vi "Event Handler.vi"(8 "error in":errorcluster, 11 "Listbox in":refnum<class "Multi Column Listbox.lvclass">) -> (0 "error out":errorcluster, 3 "Listbox out":refnum<class "Multi Column Listbox.lvclass">)   [LabVIEW 2013, in "Table Manager.lvlib" / "Multi Column Listbox.lvclass"]
doc: "Contains a loop and event structure to handle all common MCLB user interactions."
uses:
  Multi Column Listbox.lvclass
  Table Manager.lvlib
  <vilib>/Utility/miscctls.llb/LVPositionTypeDef.ctl
  Table Manager/Menu Select.ctl
  Table Manager/Table Manager.lvclass
  <vilib>/Utility/miscctls.llb/LVRowAndColumnTypeDef.ctl
panel:
  out "Char":i16
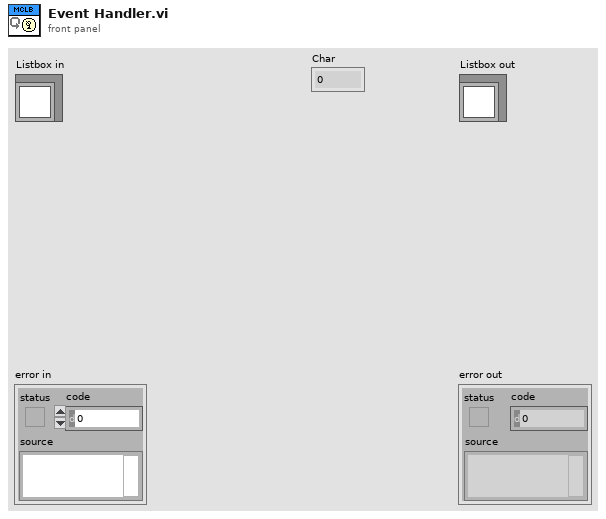
[diagram p1: front panel]
types:
  T1 = typedef "LVPositionTypeDef.ctl" = cluster{"Left":i32, "Top":i32}
  T2 = typedef "LVRowAndColumnTypeDef.ctl" = cluster{"Row":i32, "Column":i32}
  T3 = typedef "Table Manager.lvlib/Table Manager.lvclass/Menu Select.ctl" = cluster{"Line Name":string, "Selected Value":string, "Row":i32, "Column":i32, "Table Index":i32}
  T4 = typedef "Table Manager.lvlib/Table Manager.lvclass/object ref.ctl" = cluster{"engine":refnum<data-value>, "Node Ref":refnum<data-value>}
  T5 = typedef "NISE_CEF_Node.lvclass/RefreshUIEvent.ctl" = refnum<user-event>
  T6 = typedef "Table Manager.lvlib/Multi Column Listbox.lvclass/Int Reg Events.ctl" = refnum<event-registration>
  T7 = typedef "control module editor.lvclass/dialog output action.ctl" = enum16{"Tag Created", "Tag Selected", "Set Default", "disconnect"}
  T8 = typedef "LVPoint32TypeDef.ctl" = cluster{"Horizontal":i32, "Vertical":i32}
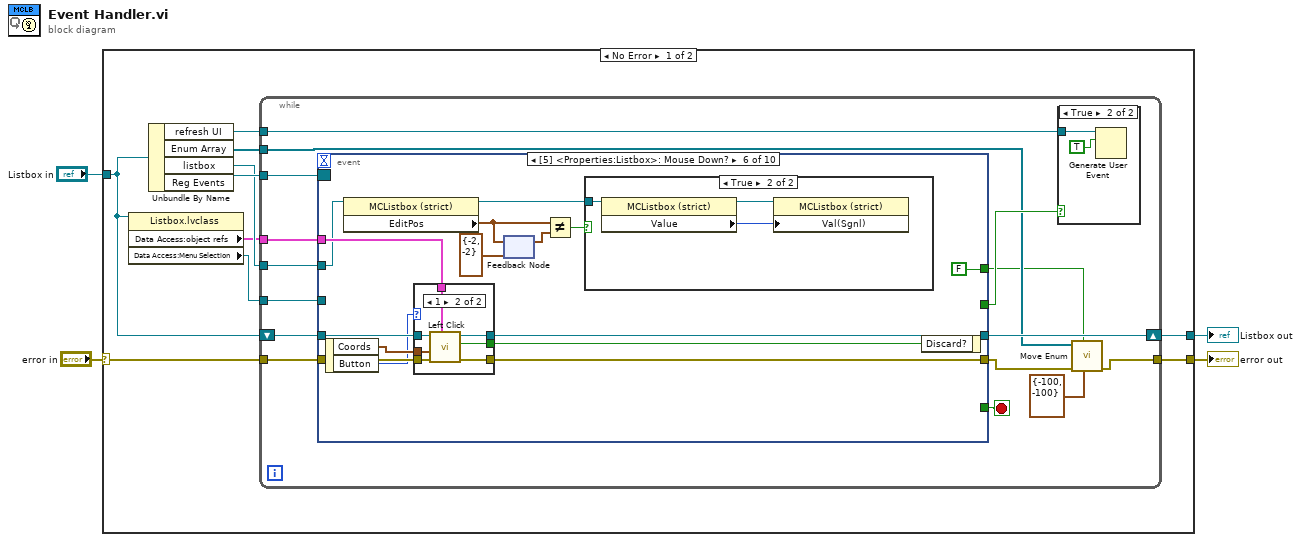
[diagram p0: block diagram]
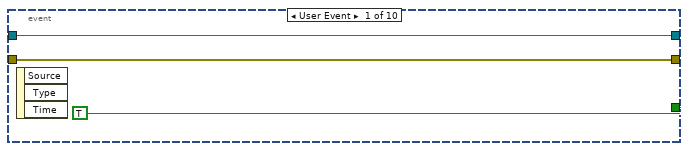
[diagram p3: hidden frame]
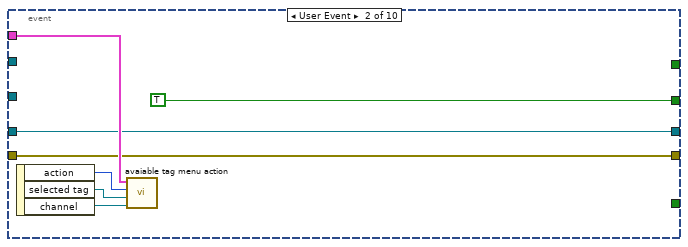
[diagram p4: hidden frame]
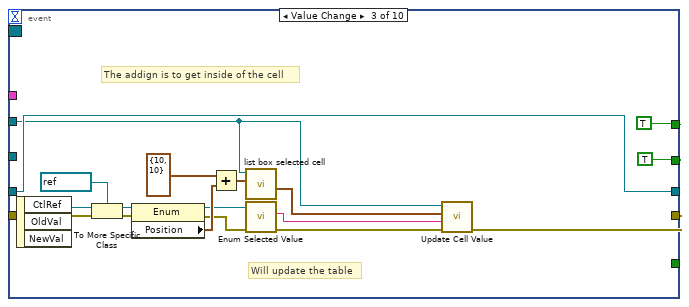
[diagram p5: hidden frame]
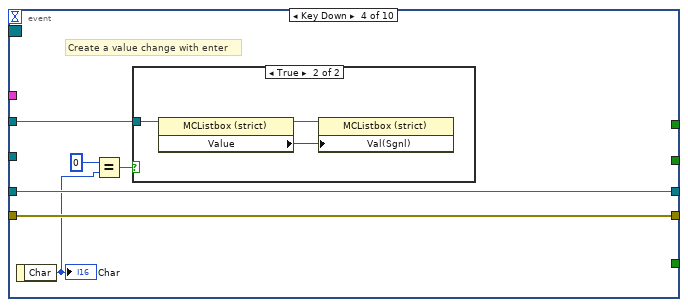
[diagram p6: hidden frame]
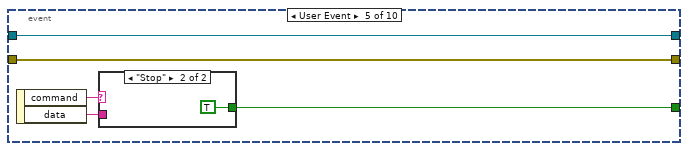
[diagram p8: hidden frame]
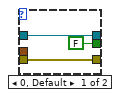
[diagram p11: hidden frame]
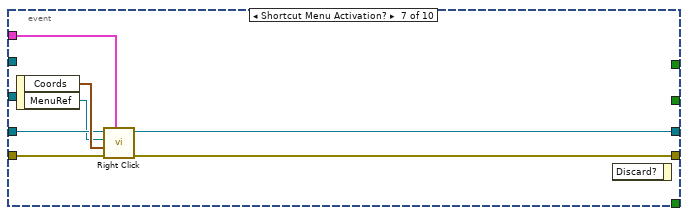
[diagram p12: hidden frame]
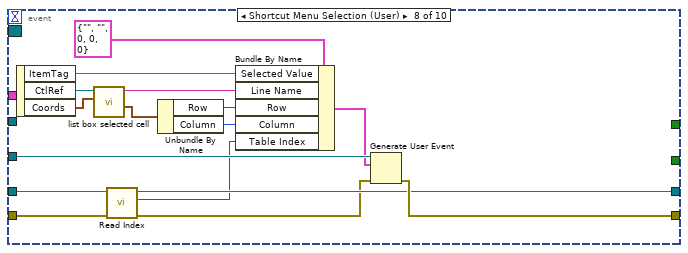
[diagram p13: hidden frame]
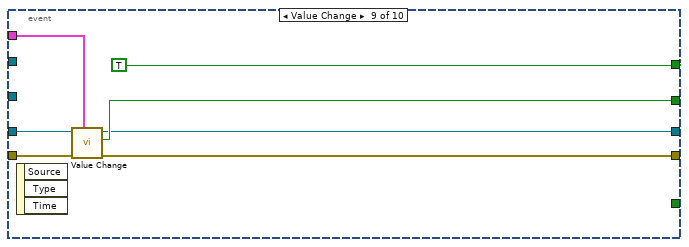
[diagram p14: hidden frame]
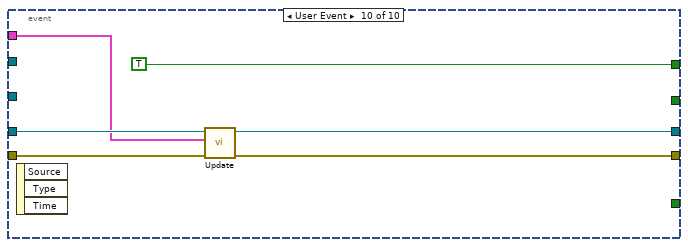
[diagram p15: hidden frame]
diagram:
  n1 = case shown="No Error" "error in" {
    selector: "error in" -> [w12 w140]
    tunnel: [w11 w140] -> w2
    tunnel: [w14 w139] -> w3
    tunnel: "Listbox in" -> [w7 w139]
    frame No Error {
      n2 = property class="Listbox.lvclass"(reference=w7) -> ("Data Access:object refs"=w6:T4, "Data Access:Menu Selection"=w5:refnum<user-event>)  [unwired: 1 in, 2 out]
      n3 = Unbundle By Name(w7) -> ("refresh UI"=w9:T5, "Enum Array"=w8:refnum<vi>[], "listbox"=w10:refnum<vi>, "Reg Events"=w13:T6)
      n4 = while {
        shift-right: [w25] -> w14
        shift-left: w7 -> [w26]
        tunnel: w13 -> [w28]
        tunnel: w6 -> [w27]
        tunnel: w12 -> [w24]
        tunnel: [w20] -> w11
        tunnel: w8 -> [w22]
        tunnel: w10 -> [w19]
        tunnel: w9 -> [w18]
        tunnel: w5 -> [w15]
        stop <- w29 stop-if-true
        n5 = event shown="[5] <Properties:Listbox>: Mouse Down?" {
          selector: w28 -> [_ _ _ _ _ _ _ _ _ _]
          dyn-events: _ -> [_ _ _ _ _ _ _ _ _ _]
          timeout: _ -> [_ _ _ _ _ _ _ _ _ _]
          tunnel: [TRUE _ _ _ w69 _ _ _ _ _] -> w29
          tunnel: w27 -> [_ w40 _ _ _ w88 w107 _ w128 w136]
          tunnel: w26 -> [w33 w39 w59 w65 w73 w83 w108 w114 w131 w138]
          tunnel: [w33 w39 w59 w65 w73 w89 w103 w113 w126 w137] -> w25
          tunnel: w24 -> [w32 w35 w48 w64 w72 w86 w106 w112 w130 w135]
          tunnel: [w32 w35 w46 w64 w72 w85 w105 w116 w129 w134] -> w21
          tunnel: [_ TRUE ("changed") TRUE ("changed") _ _ _ _ _ w127 _] -> w23
          tunnel: [_ _ TRUE _ _ FALSE _ _ TRUE TRUE] -> w16
          tunnel: w19 -> [_ _ w57 w60 _ w80 _ _ _ _]
          tunnel: w15 -> [_ _ _ _ _ _ _ w123 _ _]
          event User Event {
            n6 = event-data() -> ()  [unwired: 1 in, 3 out]
          }
          event User Event {
            n7 = event-data() -> ("action"=w41:T7, "selected tag"=w38:refnum<class "tag descriptor.lvclass">, "channel"=w37:refnum<class "TBM channel.lvclass">)  [unwired: 1 in]
            n8 = call "avaiable tag menu action.vi"("channel"=w37, "selected tag"=w38, "action"=w41, "object ref"=w40) -> ()  [unwired: 6 in, 2 out]
          }
          event Value Change {
            # "Will update the table"
            # "The addign is to get inside of the cell"
            n9 = event-data() -> ("CtlRef"=w58:refnum<vi>)  [unwired: 1 in, 2 out]
            n10 = To More Specific Class(target class=refnum<vi> refnum ("Enum"), reference=w58, error in=w48) -> (specific class reference=w44:refnum<vi>, error out=w47:errorcluster)
            n11 = property class="Enum"(reference=w44, error in=w47) -> (reference out=w43:refnum<vi>, error out=w42:errorcluster, "Position"=w52:T1)
            n12 = Add(x=T1 {"Left"=10, "Top"=10} ("y"), y=w52) -> (x+y=w50:T1)
            n13 = call "list box selected cell.vi"("Coords"=w50, "MulticolumnListbox in"=w57) -> ("cell position"=w53:T2)  [unwired: 6 in, 3 out]
            n14 = call "Enum Selected Value.vi"("error in"=w42, "Enum"=w43) -> ("error out"=w45:errorcluster, "Value"=w49:string)  [unwired: 7 in, 1 out]
            n15 = call "Update Cell Value.vi"("error in"=w45, "Value"=w49, "cell position in"=w53, "MulticolumnListbox in"=w57) -> ("error out"=w46:errorcluster)  [unwired: 6 in, 1 out]
          }
          event Key Down {
            # "Create a value change with enter"
            n16 = event-data() -> ("Char"=w63:i16)  [unwired: 1 in]
            "Char" <- w63
            n17 = Equal?(x=i16 0, y=w63) -> (x = y?=w61:bool)
            n18 = case shown="True" w61 {
              tunnel: w60 -> [_ w68]
              frame False {
              }
              frame True {
                n19 = property class="MCListbox (strict)"(reference=w68) -> (reference out=w67:refnum<vi>, "Value"=w66:i32)  [unwired: 1 in, 1 out]
                n20 = property class="MCListbox (strict)"(reference=w67, "Val(Sgnl)"=w66) -> ()  [unwired: 1 in, 2 out]
              }
            }
          }
          event User Event {
            n21 = event-data() -> ("command"=w71:string, "data"=w70:string)  [unwired: 1 in]
            n22 = case shown="\"Stop\"" w71 {
              tunnel: [_ TRUE] -> w69
              tunnel: w70 -> [_ _]
              frame Default {
              }
              frame "Stop" {
              }
            }
          }
          event Mouse Down? {
            n23 = event-data() -> ("Coords"=w87:T8, "Button"=w81:u16)  [unwired: 1 in]
            n24 = property class="MCListbox (strict)"(reference=w80) -> (reference out=w75:refnum<vi>, "EditPos"=w79:T2)  [unwired: 1 in, 1 out]
            n25 = case shown="1" w81 {
              tunnel: [w95 w102] -> w89
              tunnel: w88 -> [_ w101]
              tunnel: w87 -> [_ w100]
              tunnel: w86 -> [w93 w99]
              tunnel: [w93 w98] -> w85
              tunnel: [FALSE ("Discard?") w97] -> w84
              tunnel: w83 -> [w95 w96]
              frame 0, Default {
              }
              frame 1 {
                n26 = call-dynamic "Left Click.vi"("object refs"=w101, "error in"=w99, "Coords"=w100, "Multi Column Listbox in"=w96) -> ("error out"=w98:errorcluster, "Discard?"=w97:bool, "Multi Column Listbox out"=w102:refnum<class "Multi Column Listbox.lvclass">)  [unwired: 5 in]
              }
            }
            n27 = feedback-in #1(w79) -> ()
            n28 = feedback #1(T2 {"Row"=-2, "Column"=-2} ("EditPos")) -> (w78:T2)
            n29 = Not Equal?(x=w79, y=w78) -> (x != y?=w76:bool)
            n30 = case shown="True" w76 {
              tunnel: w75 -> [_ w92]
              frame False {
              }
              frame True {
                n31 = property class="MCListbox (strict)"(reference=w92) -> (reference out=w91:refnum<vi>, "Value"=w90:i32)  [unwired: 1 in, 1 out]
                n32 = property class="MCListbox (strict)"(reference=w91, "Val(Sgnl)"=w90) -> ()  [unwired: 1 in, 2 out]
              }
            }
            n33 = event-data("Discard?"=w84) -> ()  [unwired: 1 in, 1 out]
          }
          event Shortcut Menu Activation? {
            n34 = event-data() -> ("Coords"=w109:T8, "MenuRef"=w104:refnum<k9>)  [unwired: 1 in]
            n35 = call-dynamic "Right Click.vi"("object refs"=w107, "error in (no error)"=w106, "Coords"=w109, "Event data"=w104, "Multi Column Listbox in"=w108) -> ("error out"=w105:errorcluster, "Multi Column Listbox out"=w103:refnum<class "Multi Column Listbox.lvclass">)  [unwired: 5 in]
            n36 = event-data() -> ()  [unwired: 2 in, 1 out]
          }
          event Shortcut Menu Selection (User) {
            n37 = event-data() -> ("ItemTag"=w115:string, "CtlRef"=w125:refnum<vi>, "Coords"=w124:T8)  [unwired: 1 in]
            n38 = call "list box selected cell.vi"("Coords"=w124, "MulticolumnListbox in"=w125) -> ("cell position"=w120:T2, "tag select name"=w121:string)  [unwired: 6 in, 2 out]
            n39 = call "Read Index.vi"("error in (no error)"=w112, "Table Manager in"=w114) -> ("error out"=w111:errorcluster, "Index"=w110:i32, "Table Manager out"=w113:refnum<class "Multi Column Listbox.lvclass">)  [unwired: 7 in]
            n40 = Unbundle By Name(w120) -> ("Row"=w119:i32, "Column"=w118:i32)
            n41 = Bundle By Name(cluster=T3 {"Line Name"="", "Selected Value"="", "Row"=0, "Column"=0, "Table Index"=0} ("event data"), "Selected Value"=w115, "Line Name"=w121, "Row"=w119, "Column"=w118, "Table Index"=w110) -> (w117:T3)
            n42 = Generate User Event(user event=w123, event data cluster=w117, error in=w111) -> (error out=w116:errorcluster)  [unwired: 1 in, 1 out]
          }
          event Value Change {
            n43 = event-data() -> ()  [unwired: 1 in, 3 out]
            n44 = call-dynamic "Value Change.vi"("objects"=w128, "error in"=w130, "Multi Column Listbox in"=w131) -> ("error out"=w129:errorcluster, "Update?"=w127:bool, "Multi Column Listbox out"=w126:refnum<class "Multi Column Listbox.lvclass">)  [unwired: 6 in]
          }
          event User Event {
            n45 = event-data() -> ()  [unwired: 1 in, 3 out]
            n46 = call-dynamic "Update.vi"("error in"=w135, "object ref in"=w136, "Multi Column Listbox in"=w138) -> ("error out"=w134:errorcluster, "Multi Column Listbox out"=w137:refnum<class "Multi Column Listbox.lvclass">)  [unwired: 6 in, 1 out]
          }
        }
        n47 = case shown="True" w23 {
          tunnel: w18 -> [_ w30]
          frame False {
          }
          frame True {
            n48 = Generate User Event(user event=w30, event data cluster=TRUE ("event data")) -> ()  [unwired: 2 in, 2 out]
          }
        }
        n49 = call "Move Enum.vi"("position"=T1 {"Left"=-100, "Top"=-100}, "move?"=w16, "error in"=w21, "Enum Array"=w22) -> ("error out"=w20:errorcluster)  [unwired: 7 in]
      }
    }
    frame Error {
    }
  }
  "error out" <- w2
  "Listbox out" <- w3
